vi "__read_temp_8ch.vi"(11 "GIPB番号":string="12") -> (3 "配列":dbl[](array[numeric])=[299.21, 300.13, 300.52, 306.4, 4.153, 4.233, 16.877, 90.958])   [LabVIEW 2017]
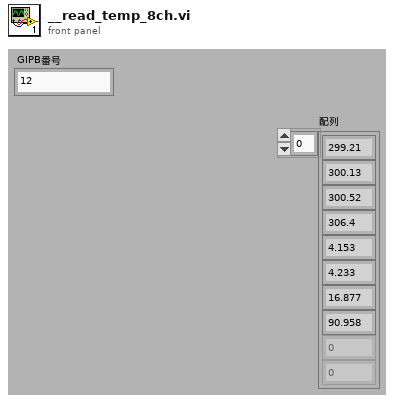
[diagram p1: front panel]
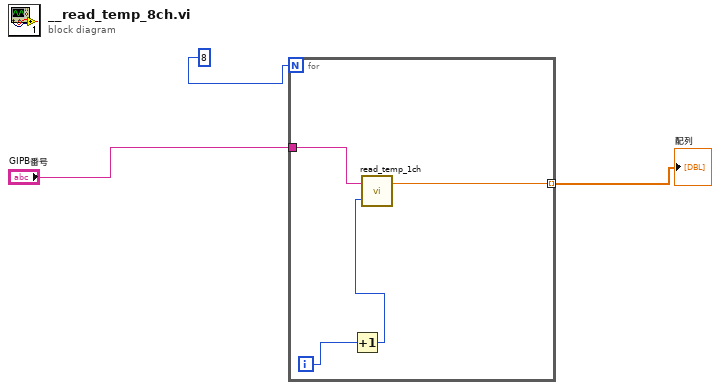
[diagram p0: block diagram]
diagram:
  n1 = for {
    N: 8 -> [_]
    tunnel: "GIPB番号" -> [w7]
    tunnel: [w4] -> w1 mode=indexing
    i -> [w6]
    n2 = Increment(x=w6) -> (x+1=w5:i32)
    n3 = call "read_temp_1ch.vi"("ch"=w5, "GIPB番号"=w7) -> ("input A"=w4:dbl)  [unwired: 1 in]
  }
  "配列" <- w1
